vi "Lambda_SubVI.vi"(0 "High Byte":u8, 3 "Low Byte":u8) -> (7 "Lambda":dbl)   [LabVIEW 2012]
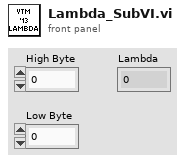
[diagram p1: front panel]
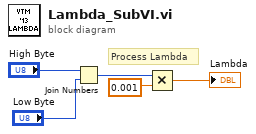
[diagram p0: block diagram]
diagram:
  # "Process Lambda"
  n1 = Join Numbers(hi="High Byte", lo="Low Byte") -> ((hi.lo)=w4:u16)
  n2 = Multiply(x=w4, y=0.001) -> (x*y=→"Lambda":dbl)
